vi "Init.vi"(8 "error in (no error)":errorcluster, 9 "SA Pin":string, 10 "Measurement Name":string) -> (0 "error out":errorcluster, 3 "CDMA2K_ModACC out":refnum<class "CDMA2K_ModACC.lvclass">)   [LabVIEW 2016, in "SeqAuto Evaluations.lvlib" / "CDMA2K_ModACC.lvclass"]
uses:
  CDMA2K_ModACC.lvclass
  C:/Sequence Automation/Plugins/SeqAuto IEvaluation.lvlibp/SeqAuto IEvaluation.lvclass
  Plugins/SeqAuto IEvaluation.lvlibp/Write Measurement Name.vi
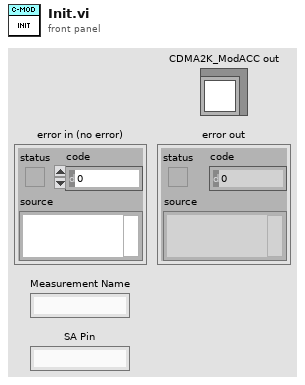
[diagram p1: front panel]
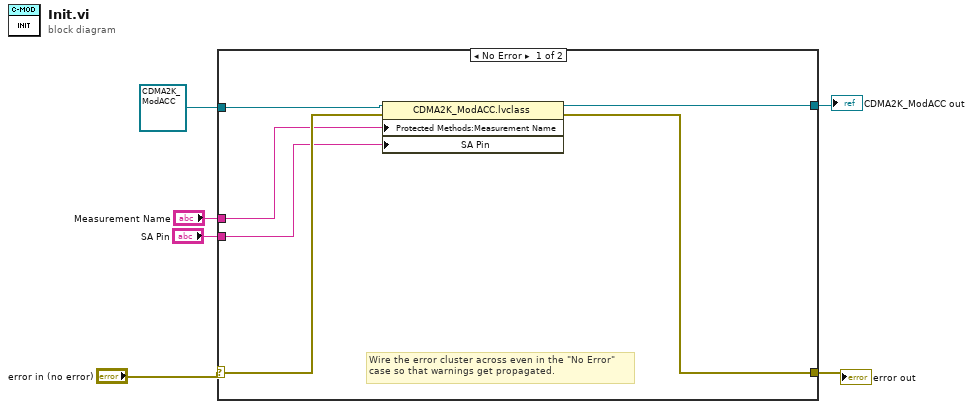
[diagram p0: block diagram]
diagram:
  n1 = case shown="No Error" "error in (no error)" {
    selector: "error in (no error)" -> [w12 w14]
    tunnel: [w11 w14] -> w2
    tunnel: "Measurement Name" -> [w10 _]
    tunnel: "SA Pin" -> [w9 _]
    tunnel: refnum<class "CDMA2K_ModACC.lvclass"> refnum ("CDMA2K_ModACC in") -> [w8 w13]
    tunnel: [w7 w13] -> w3
    frame No Error {
      # "Wire the error cluster across even in the \"No Error\"\ncase so that warnings get propagated."
      n2 = property class="CDMA2K_ModACC.lvclass"(reference=w8, error in=w12, "Protected Methods:Measurement Name"=w10, "SA Pin"=w9) -> (reference out=w7:refnum<class "CDMA2K_ModACC.lvclass">, error out=w11:errorcluster)
    }
    frame Error {
    }
  }
  "error out" <- w2
  "CDMA2K_ModACC out" <- w3
